vi "Read Refs.vi"(11 "TEMPLATE Refs in":refnum<class "TEMPLATE Refs.lvclass">) -> (2 "Refs":T1)   [LabVIEW 2025, in "_Template.lvlib" / "Templates.lvlib" / "TEMPLATE Actor.lvlib" / "TEMPLATE Refs.lvclass"]
uses:
  TEMPLATE Refs.lvclass
  Refs.ctl
  TEMPLATE Refs.lvclass/TEMPLATE Refs.ctl
  TEMPLATE Actor.lvlib
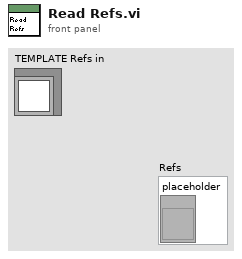
[diagram p1: front panel]
types:
  T1 = typedef "_Template.lvlib/Templates.lvlib/TEMPLATE Actor.lvlib/Refs.ctl" = cluster{"placeholder":refnum<vi>}
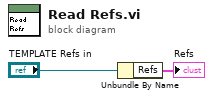
[diagram p0: block diagram]
diagram:
  n1 = Unbundle By Name("TEMPLATE Refs in") -> ("Refs"=→"Refs":T1)
